vi "pixelfly_close.vi"(1 "error in (no error)":errorcluster, 2 "Buffer number":i32, 3 "boardid in":i32) -> (0 "error out":errorcluster)   [LabVIEW 2013]
doc: "This VI stops the PixelFly camera, frees up memory (camera and buffer), and releases the camera board from computer control."
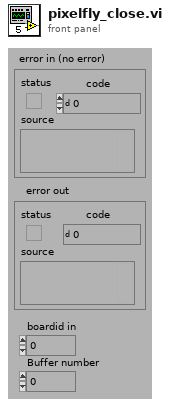
[diagram p1: front panel]
types:
  T1 = cluster{"Write":bool, "Write done":bool, "Queued":bool, "Cancelled":bool, "Select":bool, "Select done":bool, "Burst":bool, "Size":bool, "Event":bool, "Timeout":bool, "Open":i32, "Map":i32, "Exposure":i32[], "Offset":i32[], "Size":i32[], "Transfer":i32[], "Total Size":i32}
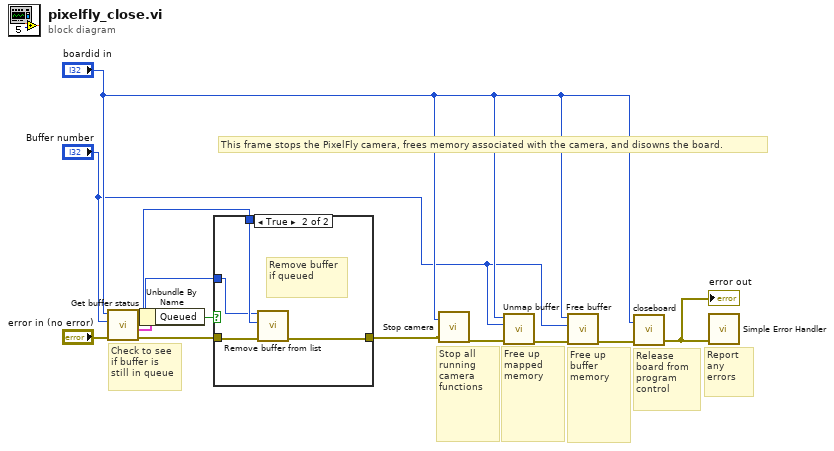
[diagram p0: block diagram]
diagram:
  # "This frame stops the PixelFly camera, frees memory associated with the camera, and disowns the board."
  # "Check to see if buffer is still in queue"
  # "Report any errors"
  # "Release board from program control"
  # "Free up buffer memory"
  # "Free up mapped memory"
  # "Stop all running camera functions"
  n1 = call "Get buffer status.vi"("error in (no error)"="error in (no error)", "Buffer request"="Buffer number", "Handle in"="boardid in") -> ("error out"=w9:errorcluster, "Buffer status"=w10:T1, "Buffer number"=w6:i32, "Handle out"=w5:i32)  [unwired: 1 in]
  n2 = Unbundle By Name(w10) -> ("Queued"=w8:bool)
  n3 = case shown="True" w8 {
    tunnel: w9 -> [w14 w18]
    tunnel: [w14 w17] -> w7
    tunnel: w6 -> [_ w16]
    tunnel: w5 -> [_ w15]
    frame False {
      # "Successfull write has removed buffer from queue"
    }
    frame True {
      # "Remove buffer if queued"
      n4 = call "Remove buffer from list.vi"("error in (no error)"=w18, "Buffer in"=w16, "Handle in"=w15) -> ("error out"=w17:errorcluster)  [unwired: 2 in, 2 out]
    }
  }
  n5 = call "Stop camera.vi"("Handle in"="boardid in", "error in (no error)"=w7) -> ("error out"=w12:errorcluster)  [unwired: 2 out]
  n6 = call "Unmap buffer.vi"("error in (no error)"=w12, "Buffer in"="Buffer number", "Handle in"="boardid in") -> ("error out"=w13:errorcluster)  [unwired: 2 in, 2 out]
  n7 = call "Free buffer.vi"("error in (no error)"=w13, "Buffer in"="Buffer number", "Handle in"="boardid in") -> ("error out"=w11:errorcluster)  [unwired: 2 in, 2 out]
  n8 = call "closeboard.vi"("Handle in"="boardid in", "error in (no error)"=w11) -> ("error out"=w4:errorcluster)  [unwired: 2 out]
  "error out" <- w4
  n9 = call <vilib>:"Simple Error Handler.vi"("error in (no error)"=w4) -> ()  [unwired: 4 in, 5 out]
